vi "CVT I32 Read.vi"(3 "error in (no error)":errorcluster, 5 "Tag Name":string) -> (0 "error out":errorcluster, 1 "Value":i32)   [LabVIEW 2010]
uses:
  Current Value Table.lvlib
  DataTypes/I32_Read.vi
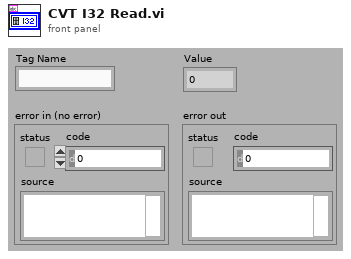
[diagram p1: front panel]
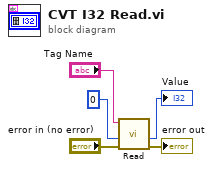
[diagram p0: block diagram]
diagram:
  n1 = call-poly "Read.vi"("error in (no error)"="error in (no error)", "Default"=0, "Tag Name"="Tag Name") -> ("error out"=→"error out":errorcluster, "Value"=→"Value":i32)  [unwired: 7 in]
